vi "StartAudioRecordingRoutedMessage_Name.vi"() -> (1 "message name":string="EmsaAudio.StartAudioRecording")   [LabVIEW 2017, in "EmsaAudio.lvlib"]
uses:
  <vilib>/addons/InsightCM/Devices/Shared/Emsa/EmsaAudio/EmsaAudio.lvlib
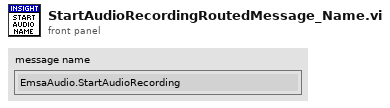
[diagram p1: front panel]
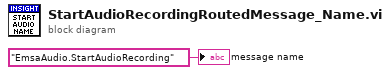
[diagram p0: block diagram]
diagram:
  "message name" <- "EmsaAudio.StartAudioRecording" ("ProcessName")
